vi "Lectura en Base de Datos.vi"() -> ()   [LabVIEW 2020]
uses:
  <vilib>/httpClient/LabVIEWHTTPClient.lvlib
panel:
  in  "stop":bool
  out "Led rele":bool
  out "Hora":string
  out "Data":string
  out "Acondicionamiento":dbl
  out "error GET":errorcluster
  out "headers GET":string
  out "body GET":string
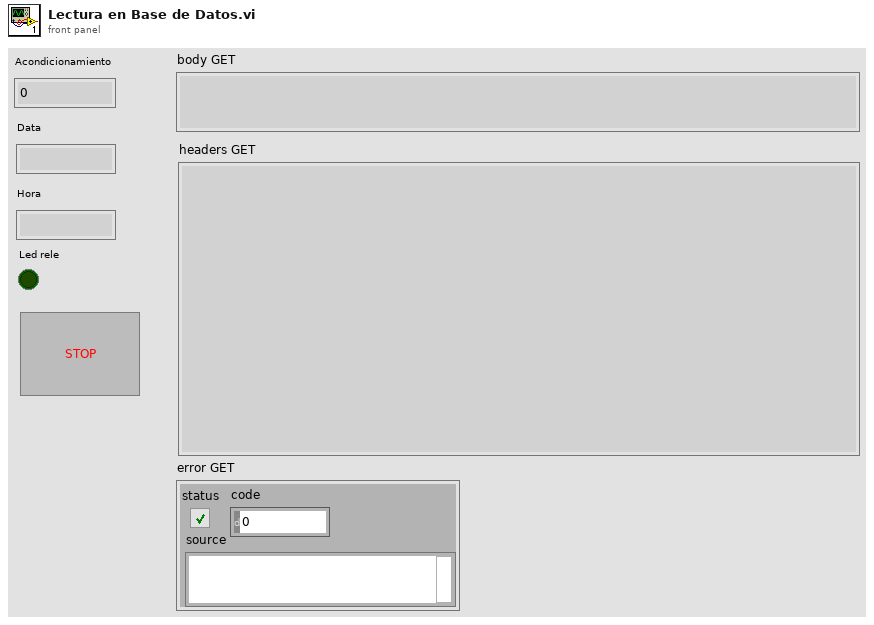
[diagram p1: front panel]
types:
  T1 = cluster{"Acondicionamiento":dbl, "Data":string, "Hora":string, "Led rele":bool}
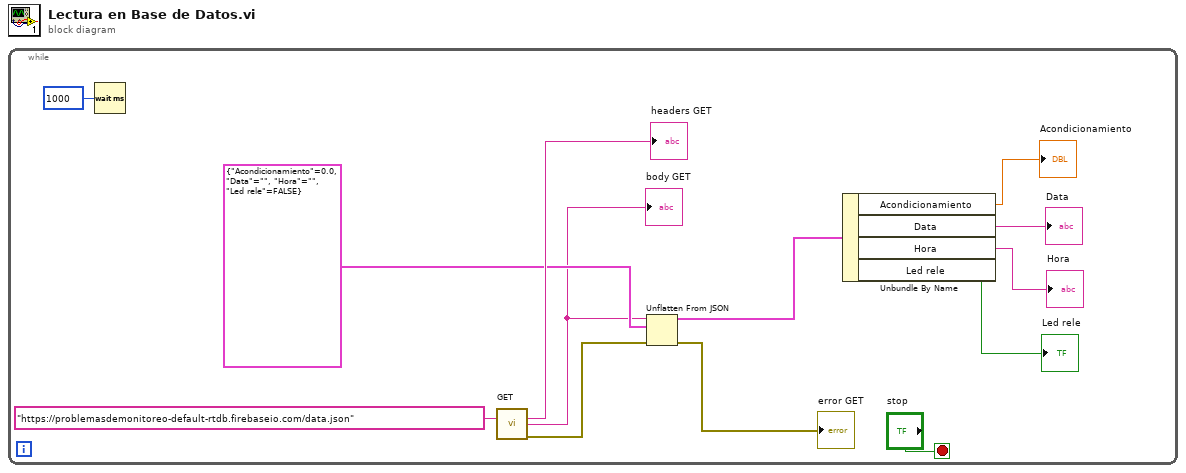
[diagram p0: block diagram]
diagram:
  n1 = while {
    stop <- "stop" stop-if-true
    n2 = Wait (ms)(milliseconds to wait=u32 1000) -> ()  [unwired: 1 out]
    n3 = call <vilib>:"GET.vi"("url"="https://problemasdemonitoreo-default-rtdb.firebaseio.com/data.json") -> ("headers"=→"headers GET":string, "body"=w1:string, "error out"=w10:errorcluster)  [unwired: 11 in, 1 out]
    "body GET" <- w1
    n4 = Unflatten From JSON(JSON string=w1, type and defaults=T1 {"Acondicionamiento"=0.0, "Data"="", "Hora"="", "Led rele"=FALSE}, error in (no error)=w10) -> (value=w9:T1, error out=→"error GET":errorcluster)  [unwired: 4 in]
    n5 = Unbundle By Name(w9) -> ("Acondicionamiento"=→"Acondicionamiento":dbl, "Data"=→"Data":string, "Hora"=→"Hora":string, "Led rele"=→"Led rele":bool)
  }
